vi "Generate Waveform.vi"(0 "signal configuration":refnum<class "SV Function.lvclass">, 5 "template waveform":waveform(dbl), 9 "samples":i32, 11 "error in (no error)":errorcluster) -> (4 "signal configuration":refnum<class "SV Function.lvclass">, 6 "output waveform":waveform(dbl), 10 "samples":i32, 15 "error out":errorcluster)   [LabVIEW 2017, in "SV Function.lvclass"]
uses:
  <vilib>/addons/_NISVFA/_Generation/Signal Generation/SV Function/SV Function.lvclass
  C:/Program Files (x86)/National Instruments/LabVIEW 2017/vi.lib/addons/_NISVFA/_Generation/Signal Generation/SV Signal/SV Signal.lvclass
  <vilib>/addons/_NISVFA/_Generation/Signal Generation/SV Signal/sv_Signal State Attribute.ctl
  <vilib>/addons/_NISVFA/_Generation/Signal Generation/SV Function/SV Function.lvclass/SV Function.ctl
  <vilib>/addons/_NISVFA/_Generation/Signal Generation/SV Signal/Read Sample Rate.vi
  <vilib>/Analysis/NI_AALBase.lvlib
  <vilib>/addons/_NISVFA/_Generation/Signal Generation/SV Signal/SV Signal.lvclass
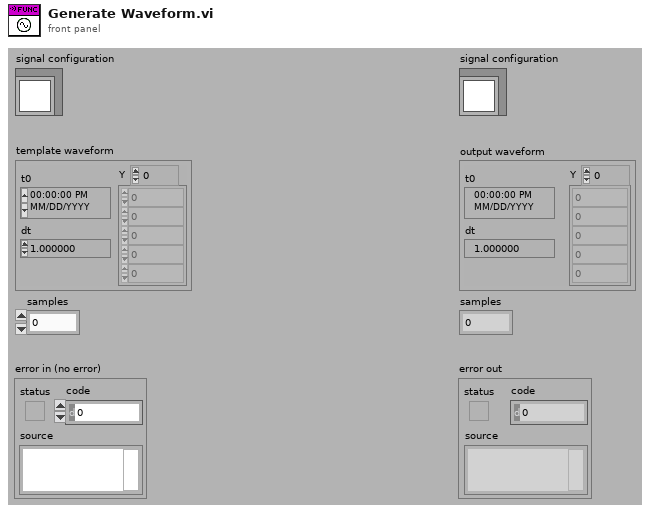
[diagram p1: front panel]
types:
  T1 = typedef "SV Signal.lvclass/sv_Signal State Attribute.ctl" = string
  T2 = typedef "SV Signal.lvclass/sv_System Timing Model.ctl" = i64
  T3 = typedef "SV Signal.lvclass/sv_Generation State.ctl" = enum16{"Idle", "Ramp Up", "Pre-Measurement Settling", "Measurement", "Post-Measurement Settling", "Discrete Sweep Transition", "Ramp Down", "Update"}
  T4 = cluster{"system timing model":T2, "state":cluster{"RESET":bool, "generator timestamp":timestamp, "elapsed seconds":dbl, "elapsed samples":u64, "generation state":T3, "time offset at state":dbl, "samples generated at state":u64, "signal state":variant}, "duration of state":dbl, "samples remaining at state":i32}
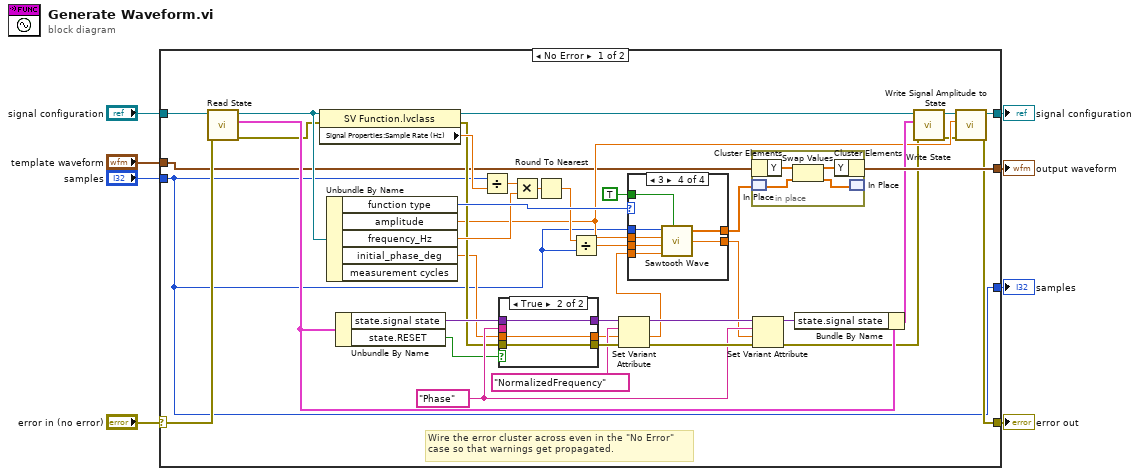
[diagram p0: block diagram]
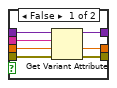
[diagram p2: hidden frame]
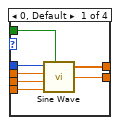
[diagram p3: hidden frame]
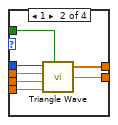
[diagram p4: hidden frame]
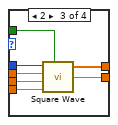
[diagram p5: hidden frame]
diagram:
  n1 = case shown="No Error" "error in (no error)" {
    selector: "error in (no error)" -> [w14 w91]
    tunnel: [w13 w91] -> w7
    tunnel: [w19 w90] -> w5
    tunnel: "signal configuration" -> [w12 w90]
    tunnel: [w38 w89] -> w4
    tunnel: [w10 _] -> w3
    tunnel: "samples" -> [w10 _]
    tunnel: "template waveform" -> [w11 w89]
    frame No Error {
      w29 = T1 "Phase" ("name")
      # "Wire the error cluster across even in the \"No Error\"\ncase so that warnings get propagated."
      n2 = call <vilib>:"Read State.vi"("error in (no error)"=w14, "signal configuration"=w12) -> ("error out"=w26:errorcluster, "generator state"=w27:T4, "signal configuration"=w28:refnum<class "SV Function.lvclass">)  [unwired: 7 in]
      n3 = property class="SV Function.lvclass"(reference=w28, error in=w26) -> (reference out=w21:refnum<class "SV Function.lvclass">, error out=w25:errorcluster, "Signal Properties:Sample Rate (Hz)"=w37:dbl)
      n4 = Unbundle By Name(w28) -> ("function type"=w46:u16, "amplitude"=w17:dbl, "frequency_Hz"=w42:dbl, "initial_phase_deg"=w24:dbl)  [unwired: 1 out]
      n5 = Unbundle By Name(w27) -> ("state.signal state"=w33:variant, "state.RESET"=w9:bool)
      n6 = Divide(x=w10, y=w37) -> (x/y=w40:dbl)
      n7 = case shown="True" w9 {
        tunnel: w33 -> [w53 w55]
        tunnel: w24 -> [w52 w56]
        tunnel: [w51 w56] -> w22
        tunnel: [w50 w55] -> w34
        tunnel: w25 -> [w49 w54]
        tunnel: [w48 w54] -> w36
        tunnel: w29 -> [w47 _]
        frame False {
          n8 = Get Variant Attribute(Variant=w53, name=w47, default value (empty Variant)=w52, error in=w49) -> (duplicate Variant=w50:variant, value=w51:dbl, error out=w48:errorcluster)  [unwired: 1 out]
        }
        frame True {
        }
      }
      n9 = Multiply(x=w40, y=w42) -> (x*y=w41:dbl)
      n10 = Round To Nearest(number=w41) -> (nearest integer value=w39:dbl)
      n11 = Divide(x=w39, y=w10) -> (x/y=w43:dbl)
      n12 = Set Variant Attribute(Variant=w34, name=T1 "NormalizedFrequency", value=w22, error in=w36) -> (Variant out=w32:variant, error out=w30:errorcluster)  [unwired: 1 out]
      n13 = case shown="3" w46 {
        tunnel: w10 -> [w63 w70 w77 w84]
        tunnel: w43 -> [w62 w69 w76 w83]
        tunnel: [w61 w68 w75 w82] -> w45
        tunnel: w17 -> [w60 w67 w74 w81]
        tunnel: w22 -> [w59 w66 w73 w80]
        tunnel: TRUE ("reset phase") -> [w58 w65 w72 w79]
        tunnel: [w57 w64 w71 w78] -> w23
        frame 0, Default {
          n14 = call <vilib>:"Sine Wave.vi"("samples"=w63, "amplitude"=w60, "frequency"=w62, "phase in"=w59, "reset phase"=w58) -> ("sine wave"=w61:dbl[], "phase out"=w57:dbl)  [unwired: 1 out]
        }
        frame 1 {
          n15 = call <vilib>:"Triangle Wave.vi"("samples"=w70, "amplitude"=w67, "frequency"=w69, "phase in"=w66, "reset phase"=w65) -> ("triangle wave"=w68:dbl[], "phase out"=w64:dbl)  [unwired: 1 out]
        }
        frame 2 {
          n16 = call <vilib>:"Square Wave.vi"("samples"=w77, "reset phase"=w72, "amplitude"=w74, "frequency"=w76, "phase in"=w73) -> ("square wave"=w75:dbl[], "phase out"=w71:dbl)  [unwired: 1 in, 1 out]
        }
        frame 3 {
          n17 = call <vilib>:"Sawtooth Wave.vi"("samples"=w84, "amplitude"=w81, "frequency"=w83, "phase in"=w80, "reset phase"=w79) -> ("sawtooth wave"=w82:dbl[], "phase out"=w78:dbl)  [unwired: 1 out]
        }
      }
      n18 = in-place {
        n19 = in-place-cluster #1(w11) -> ("Y"=w88:dbl[])
        n20 = in-place-match #2(w45) -> (w86:dbl[])
        n21 = Swap Values(12:w88, 14:w86) -> (1:w87:dbl[], 3:w85:dbl[])  [unwired: 1 in]
        n22 = in-place-cluster #1("Y"=w87) -> (w38:waveform(dbl))
        n23 = in-place-match #2(w85) -> ()  [unwired: 1 out]
      }
      n24 = Set Variant Attribute(Variant=w32, name=w29, value=w23, error in=w30) -> (Variant out=w31:variant, error out=w16:errorcluster)  [unwired: 1 out]
      n25 = Bundle By Name(cluster=w27, "state.signal state"=w31) -> (w18:T4)
      n26 = call <vilib>:"Write State.vi"("error in (no error)"=w16, "generator state"=w18, "signal configuration"=w21) -> ("error out"=w15:errorcluster, "signal configuration"=w20:refnum<class "SV Function.lvclass">)  [unwired: 7 in]
      n27 = call <vilib>:"Write Signal Amplitude to State.vi"("error in (no error)"=w15, "amplitude"=w17, "SV Signal in"=w20) -> ("error out"=w13:errorcluster, "SV Signal out"=w19:refnum<class "SV Function.lvclass">)  [unwired: 7 in]
    }
    frame Error {
    }
  }
  "error out" <- w7
  "signal configuration" <- w5
  "output waveform" <- w4
  "samples" <- w3
